vi "Obtain Message Queue.vi"(7 "max queue size (-1, unlimited)":i32, 8 "error in (no error)":errorcluster, 11 "VI Reference":refnum<vi>) -> (0 "error out":errorcluster, 3 "Event Registration Refnum":refnum<event-registration>)   [LabVIEW 2020, in "COnfiguration Database.lvlib"]
doc: "Create a queue with the Message Cluster data type."
uses:
  COnfiguration Database.lvlib
  Private Controls/Message Cluster.ctl
  Private Controls/Message enum.ctl
  Private Controls/FG Actions.ctl
  Support/Stop User Event/Controls/User event Actions.ctl
  Support/Stop User Event/User Event - Stop.lvlib
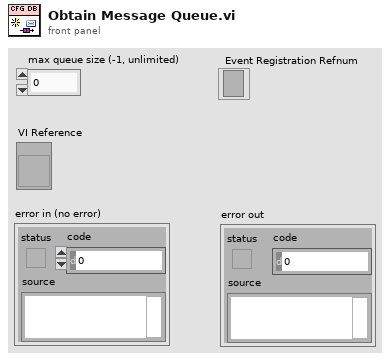
[diagram p1: front panel]
types:
  T1 = typedef "User Event - Stop.lvlib/User event Actions.ctl" = enum16{"Create", "Get Reference", "Fire Stop Event", "Destroy"}
  T2 = typedef "COnfiguration Database.lvlib/FG Actions.ctl" = enum16{"Get", "Set", "Clear"}
  T3 = typedef "COnfiguration Database.lvlib/Message Cluster.ctl" = cluster{"Message":T4, "Data":variant}
  T4 = typedef "COnfiguration Database.lvlib/Message enum.ctl" = enum16{"Initialize", "State", "Error", "Exit"}
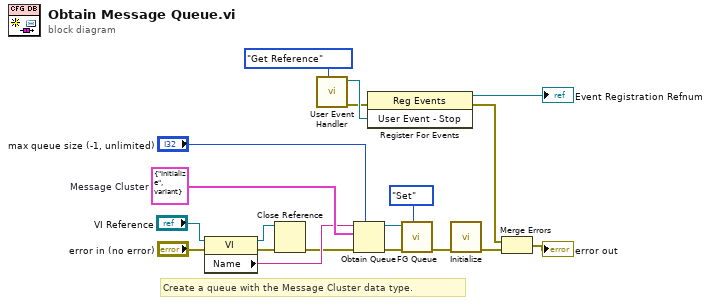
[diagram p0: block diagram]
diagram:
  w18 = T3 {"Message"=enum."Initialize", "Data"=variant}  # Message Cluster
  # "Create a queue with the Message Cluster data type."
  n1 = property class="VI"(reference="VI Reference", error in="error in (no error)") -> (reference out=w10:refnum<vi>, error out=w13:errorcluster, "Name"=w12:string)
  n2 = Close Reference(reference=w10, error in (no error)=w13) -> (error out=w11:errorcluster)
  n3 = call "User Event Handler.vi"("User Event Action"=User_event_Actions."Get Reference") -> ("error out"=w3:errorcluster, "User Event - Stop"=w7:refnum<user-event>)  [unwired: 9 in]
  n4 = Obtain Queue(max queue size (-1, unlimited)="max queue size (-1, unlimited)", name (unnamed)=w12, element data type=w18, error in (no error)=w11) -> (queue out=w16:refnum<queue>, error out=w15:errorcluster)  [unwired: 1 in, 1 out]
  n5 = register-events(error in=w3, w7) -> (reference out=→"Event Registration Refnum":refnum<event-registration>, error out=w5:errorcluster)  [unwired: 1 in]
  n6 = call "FG Queue.vi"("FG Actions"=FG_Actions."Set", "error in (no error)"=w15, "Message Queue"=w16) -> ("error out"=w2:errorcluster)  [unwired: 7 in, 1 out]
  n7 = call "Initialize.vi"("error in (no error)"=w2) -> ("error out"=w1:errorcluster)  [unwired: 10 in]
  n8 = Merge Errors(w5, w1) -> (→"error out":errorcluster)
